vi "MAG ON.vi"(8 "error in (no error)":errorcluster, 9 "PSU Status In":T1 {"Trip Current" format="%.3f"; "Trip Field" format="%.4f"; "Voltage" format="%.2f"; "Field Constant" format="%.6f"; "MID Setpoint (T)" format="%.4f"; "MID Setpoint (A)" format="%.3f"; "MAX Setpoint (T)" format="%.4f"; "MAX Setpoint (A)" format="%.3f"; "Heater Voltage" format="%.2f"; "V Limit (V)" format="%.2f"; "Ramp Rate (A/s)" format="%.3f"; "Output (A)" format="%.3f"; "Output (T)" format="%.4f"; "Persistent Current" format="%.3f"; "Persistent Field" format="%.4f"}, 10 "MagQ in":refnum<queue>, 11 "VISA Refnum in":refnum<visa-resource-name>) -> (0 "error out":errorcluster, 1 "PSU Status Out":T1 {"Trip Current" format="%.3f"; "Trip Field" format="%.4f"; "Voltage" format="%.2f"; "Field Constant" format="%.6f"; "MID Setpoint (T)" format="%.4f"; "MID Setpoint (A)" format="%.3f"; "MAX Setpoint (T)" format="%.4f"; "MAX Setpoint (A)" format="%.3f"; "Heater Voltage" format="%.2f"; "V Limit (V)" format="%.2f"; "Ramp Rate (A/s)" format="%.3f"; "Output (A)" format="%.3f"; "Output (T)" format="%.4f"; "Persistent Current" format="%.3f"; "Persistent Field" format="%.4f"}, 2 "MagQ out":refnum<queue>, 3 "VISA Refnum out":refnum<visa-resource-name>, 5 "MID Setpoint (T)":dbl)   [LabVIEW 2025]
uses:
  <instrlib>/SMS LabVIEW Drivers/Source Code/Public/PSU Status.ctl
  <instrlib>/SMS LabVIEW Drivers/Source Code/Cryogenic Ltd SMSXXX.lvlib
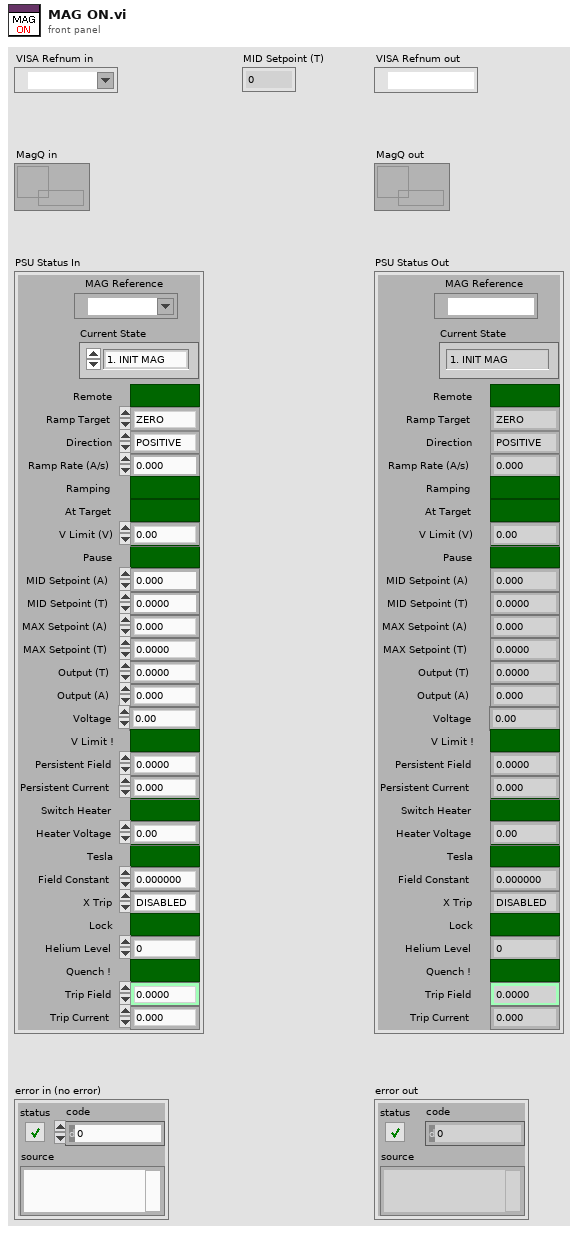
[diagram p1: front panel]
types:
  T1 = typedef "PSU Status.ctl" = cluster{"Ramp Target":enum16{"ZERO", "MID", "MAX"}, "Pause":bool, "Switch Heater":bool, "Persistent Field":dbl, "Persistent Current":dbl, "Tesla":bool, "Output (T)":dbl, "Output (A)":dbl, "X Trip":enum16{"DISABLED", "ENABLED", "ACTIVE"}, "Ramp Rate (A/s)":dbl, "V Limit (V)":dbl, "Heater Voltage":dbl, "MAX Setpoint (A)":dbl, "MAX Setpoint (T)":dbl, "MID Setpoint (A)":dbl, "MID Setpoint (T)":dbl, "Lock":bool, "Field Constant":dbl, "Remote":bool, "Direction":enum16{"POSITIVE", "NEGATIVE", "OPEN", "UNIPOLAR"}, "Helium Level":u16, "Quench !":bool, "Voltage":dbl, "V Limit !":bool, "Ramping":bool, "At Target":bool, "Trip Field":dbl, "Trip Current":dbl, "Current State":enum16{"1. INIT MAG", "2. MAG ON", "3. MAG_STAB", "4. MAG IDLE", "5. PREP NEXT FIELD", "6. APPLY NEXT FIELD", "7. PREP OFF", "8. MAG OFF (Reset)"}, "MAG Reference":refnum<visa-resource-name>}
  T2 = enum16{"1. INIT MAG", "2. MAG ON", "3. MAG_STAB", "4. MAG IDLE", "5. PREP NEXT FIELD", "6. APPLY NEXT FIELD", "7. PREP OFF", "8. MAG OFF (Reset)"}
  T3 = enum16{"RAMP TO ZERO", "RAMP TO MID", "RAMP TO MAX"}
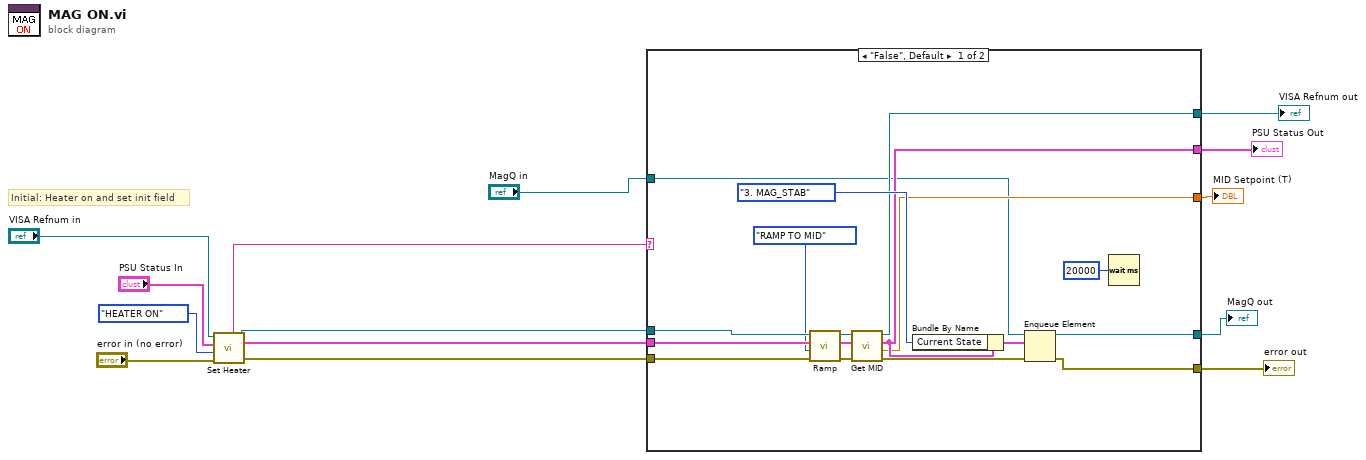
[diagram p0: block diagram]
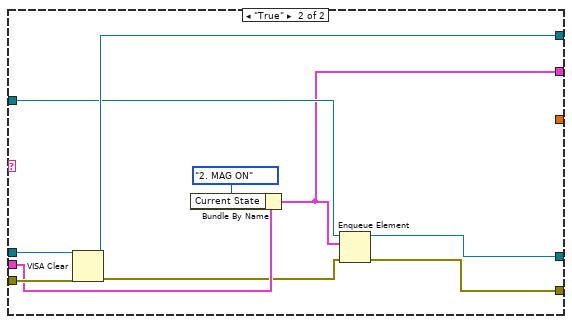
[diagram p2: hidden frame]
diagram:
  # "Initial: Heater on and set init field"
  n1 = call <instrlib>:"Set Heater.vi"("Error in (no error)"="error in (no error)", "Heater (On/Off)"=enum16{"HEATER OFF", "HEATER ON"}."HEATER ON", "PSU Status In"="PSU Status In", "VISA Resource Name In"="VISA Refnum in") -> ("Error out"=w12:errorcluster, "PSU Status Out"=w13:T1, "VISA Resource Name Out"=w11:refnum<visa-resource-name>, "Answer"=w7:string)  [unwired: 4 in]
  n2 = case shown="\"False\", Default" w7 {
    tunnel: w13 -> [w28 w38]
    tunnel: w12 -> [w27 w40]
    tunnel: w11 -> [w26 w41]
    tunnel: [w21 w35] -> w6
    tunnel: [w20 w34] -> w5
    tunnel: [w19 w39] -> w4
    tunnel: [w18 w32] -> w3
    tunnel: [w17 _] -> w2
    tunnel: "MagQ in" -> [w16 w36]
    frame "False", Default {
      n3 = call <instrlib>:"Ramp.vi"("Error in (no error)"=w27, "Ramp Target"=T3."RAMP TO MID", "PSU Status In"=w28, "VISA Resource Name In"=w26) -> ("Error out"=w25:errorcluster, "PSU Status Out"=w24:T1, "VISA Resource Name Out"=w23:refnum<visa-resource-name>)  [unwired: 4 in, 1 out]
      n4 = call <instrlib>:"Get MID.vi"("Error in (no error)"=w25, "PSU Status In"=w24, "VISA Resource Name In"=w23) -> ("Error out"=w30:errorcluster, "MID Setpoint (T)"=w17:dbl, "PSU Status Out"=w18:T1, "VISA Resource Name Out"=w19:refnum<visa-resource-name>)  [unwired: 3 in, 2 out]
      n5 = Bundle By Name(cluster=w18, "Current State"=T2."3. MAG_STAB") -> (w29:T1)
      n6 = Enqueue Element(queue=w16, element=w29, error in (no error)=w30) -> (queue out=w21:refnum<queue>, error out=w20:errorcluster)  [unwired: 1 in, 1 out]
      n7 = Wait (ms)(milliseconds to wait=u32 20000) -> ()  [unwired: 1 out]
    }
    frame "True" {
      n8 = VISA Clear(VISA resource name=w41, error in (no error)=w40) -> (VISA resource name out=w39:refnum<visa-resource-name>, error out=w33:errorcluster)
      n9 = Bundle By Name(cluster=w38, "Current State"=T2."2. MAG ON") -> (w32:T1)
      n10 = Enqueue Element(queue=w36, element=w32, error in (no error)=w33) -> (queue out=w35:refnum<queue>, error out=w34:errorcluster)  [unwired: 1 in, 1 out]
    }
  }
  "MagQ out" <- w6
  "error out" <- w5
  "VISA Refnum out" <- w4
  "PSU Status Out" <- w3
  "MID Setpoint (T)" <- w2
